vi "TrajCurrToPrev.vi"(8 "error in (no error)":errorcluster, 11 "ForceField":refnum<class "ForceField.lvclass">) -> (0 "error out":errorcluster, 1 "AnkleTraj_array":dbl[][](array[numeric]), 2 "AnkleTraj":T1[](array[typedef]), 3 "ForceField 2":refnum<class "ForceField.lvclass">)   [LabVIEW 2015, in "ForceField.lvclass"]
uses:
  ForceField.lvclass
  TypeDef/AnkleTrajPt.ctl
  ForceField.lvclass/ForceField.ctl
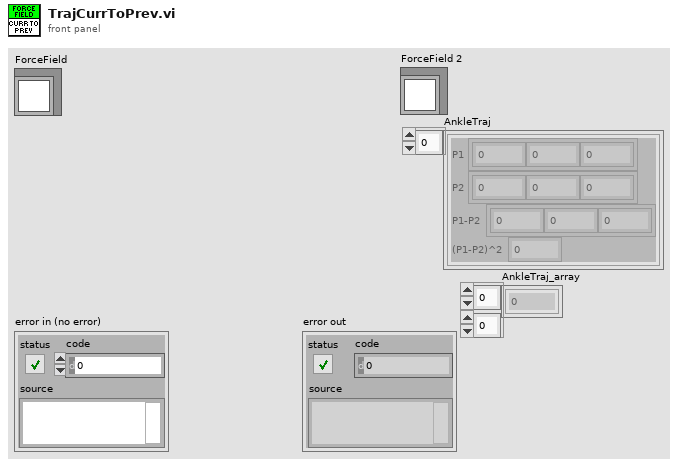
[diagram p1: front panel]
types:
  T1 = typedef "ForceField.lvclass/AnkleTrajPt.ctl" = cluster{"P1":dbl[], "P2":dbl[], "P1-P2":dbl[], "(P1-P2)^2":dbl}
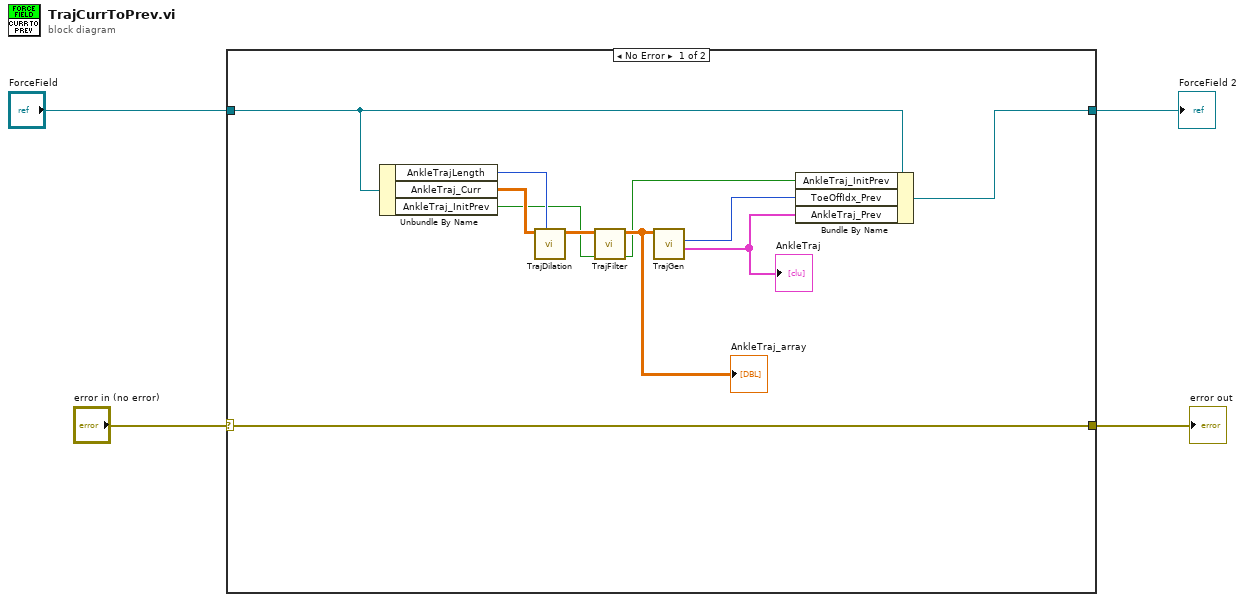
[diagram p0: block diagram]
diagram:
  n1 = case shown="No Error" "error in (no error)" {
    selector: "error in (no error)" -> [w5 w17]
    tunnel: [w5 w17] -> w3
    tunnel: "ForceField" -> [w9 w16]
    tunnel: [w8 w16] -> w1
    frame No Error {
      n2 = Unbundle By Name(w9) -> ("AnkleTrajLength"=w13:i32, "AnkleTraj_Curr"=w12:dbl[][], "AnkleTraj_InitPrev"=w11:bool)
      n3 = call "TrajDilation.vi"("Length"=w13, "TrajBeforeDilation"=w12) -> ("TrajAfterDilation"=w15:dbl[][])  [unwired: 9 in]
      n4 = call "TrajFilter.vi"("AnkleTraj_Init"=w11, "CurrentTraj"=w15) -> ("AnkleTraj_Init 2"=w10:bool, "AverageTraj"=w14:dbl[][])  [unwired: 6 in]
      "AnkleTraj_array" <- w14
      n5 = call "TrajGen.vi"("AnkleTraj"=w14) -> ("AnkleTraj"=w6:T1[], "ToeOffIdx"=w7:i32)  [unwired: 5 in, 2 out]
      "AnkleTraj" <- w6
      n6 = Bundle By Name(cluster=w9, "AnkleTraj_InitPrev"=w10, "ToeOffIdx_Prev"=w7, "AnkleTraj_Prev"=w6) -> (w8:refnum<class "ForceField.lvclass">)
    }
    frame Error {
    }
  }
  "error out" <- w3
  "ForceField 2" <- w1
